vi "LJStreamUD.vi"() -> ()   [LabVIEW 2021]
uses:
  sub/LJstreamUD globals.vi
panel:
  in  "Change Working Directory":bool
  in  "SettlingFactor":i32
  in  "Resolution":i32=1
  in  "Max File Size (Bytes)":i32=1048576 min=1 max=2000000000
  in  "Graph?":bool[](array[boolean])
  out "Address":string
  in  "Disable Scaling":bool
  out "Device Type":string
  in  "stop stream":bool
  in  "exit":bool
  in  "Graph History":i32=1000 min=0
  out "Channel Config":T1={"# Channels"=4, "+Ch"=["0", "1", "2", "3", "4", "5", "6", "7"], "-Ch (U3)"=["31", "31", "31", "31", "31", "31", "31", "31"], "Ranges (UE9)"=[0, 0, 0, 0, 0, 0, 0, 0], "Scaling Equation"=["y=v0", "y=v1", "y=v2", "y=v3", "y=v4", "y=v5", "y=v6", "y=v7"]} {"Ranges (UE9)" items=["LJ_rgBIP5V", "LJ_rgUNI5V", "LJ_rgUNI2P5V", "LJ_rgUNI1P25V", "LJ_rgUNIP625V"]}
  out "Scaled":dbl[](array[numeric]) format="%.6f"
  in  "Scaling Equation":string[](array[string])=["y=v0", "y=v1", "y=v2", "y=v3", "y=v4", "y=v5", "y=v6", "y=v7"]
  in  "# Channels":i32=4 min=1
  in  "-Ch":string[](array[string])=["199", "199", "199", "199", "199", "199", "199", "199"]
  out "Voltage":dbl[](array[numeric]) format="%.6f"
  in  "Ranges":u16[](array[ring])=[0, 0, 0, 0, 0, 0, 0, 0] items=["LJ_rgBIP10V", "LJ_rgBIP5V", "LJ_rgUNI5V", "LJ_rgUNI2P5V", "LJ_rgUNI1P25V", "LJ_rgBIP1V", "LJ_rgUNIP625V", "LJ_rgBIPP1V", "LJ_rgBIPP01V"]
  out "Waveform Graph":cluster{dbl, dbl, dbl[][]}(graph)
  out "UD Backlog [%]":dbl format="%.2f"
  in  "+Ch":string[](array[string])=["0", "1", "2", "3", "4", "5", "6", "7"]
  out "ms Per Loop":u32
  out "Device Backlog [%]":dbl format="%.2f"
  out "# Scans Read":i32
  out "# of iterations":i32
  in  "Scan Rate (Hz)":dbl=500.0 format="%.3f"
  out "Current Data File":path
  in  "Data File Prefix":string="data"
  in  "Write To File":bool
  in  "start stream":bool caption="Start Stream"
  out "Last Stream Error Message":string
  # "0"
  # "1"
  # "2"
  # "3"
  # "4"
  # "5"
  # "6"
  # "7"
  # "8"
  # "9"
  # "10"
  # "11"
  # "12"
  # "13"
  # "14"
  # "15"
  # "Scaling is computing intensive.  If UD Backlog\n  is growing, disable scaling."
  # "# scans"
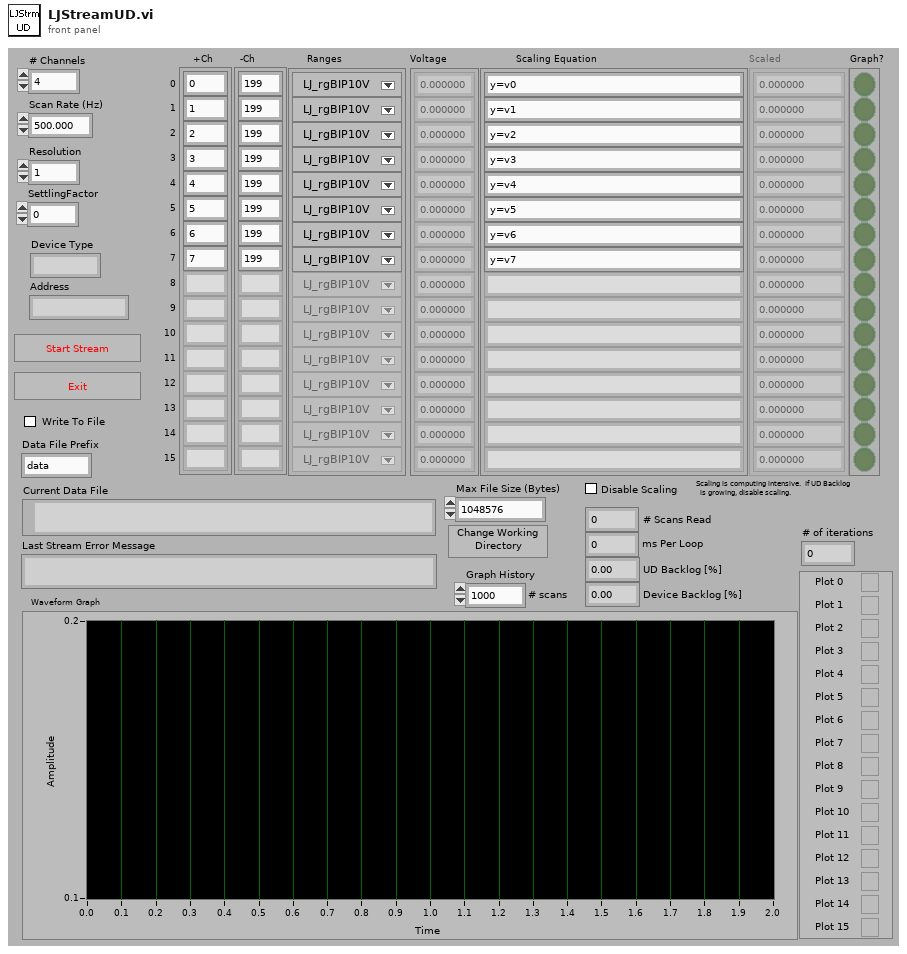
[diagram p1: front panel]
types:
  T1 = cluster{"# Channels":i32, "+Ch":string[], "-Ch (U3)":string[], "Ranges (UE9)":u16[], "Scaling Equation":string[]}
  T2 = cluster{"+Ch":string[], "-Ch":string[], "Ranges":u16[], "Scaling Equation":string[], "Graph?":bool[]}
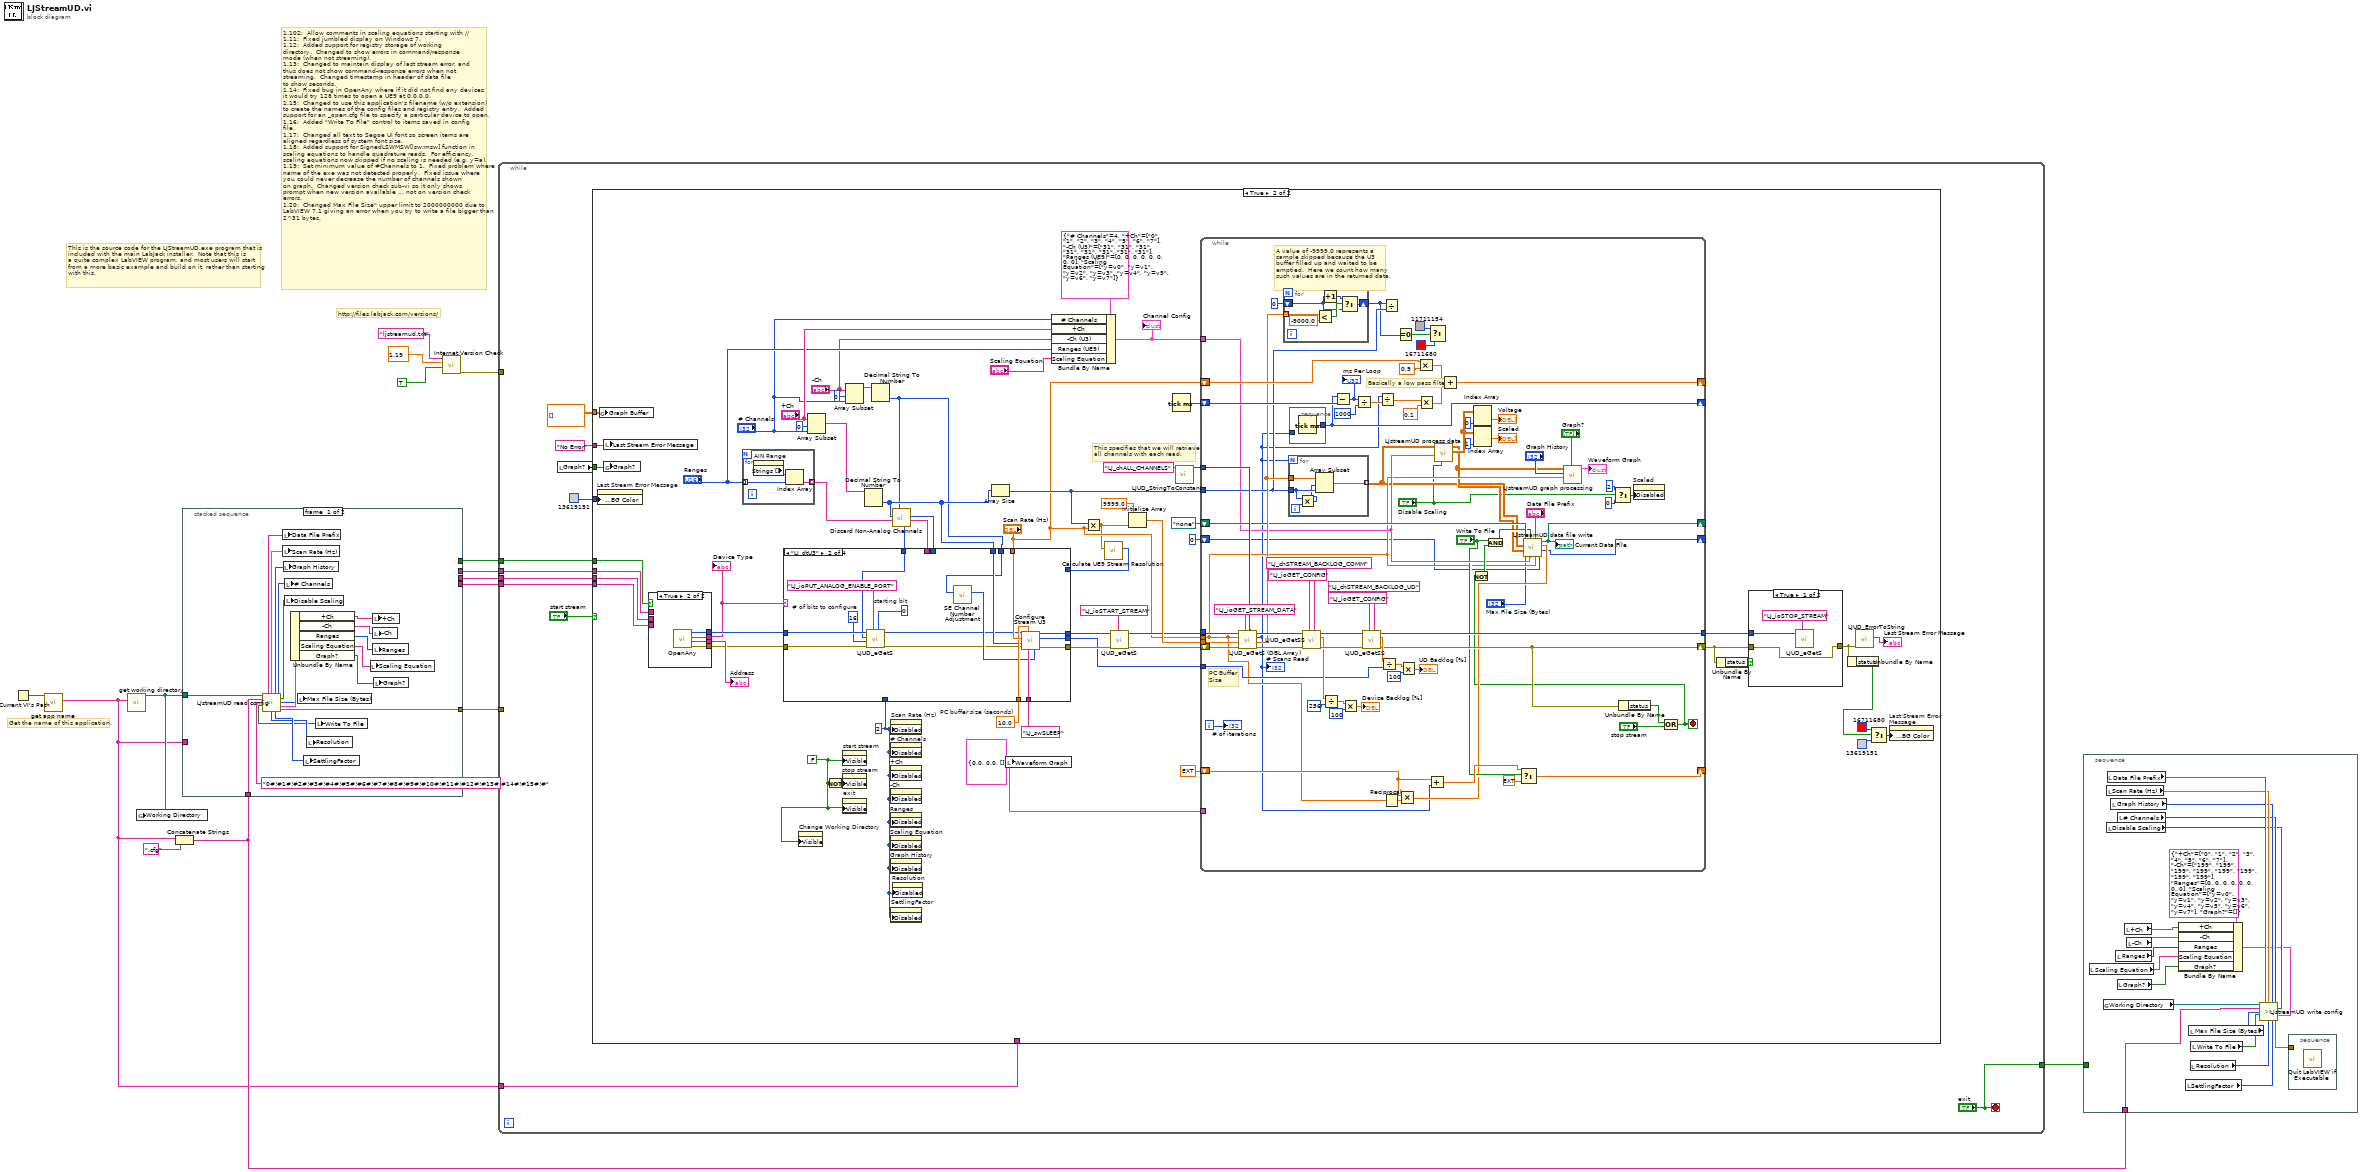
[diagram p0: block diagram]
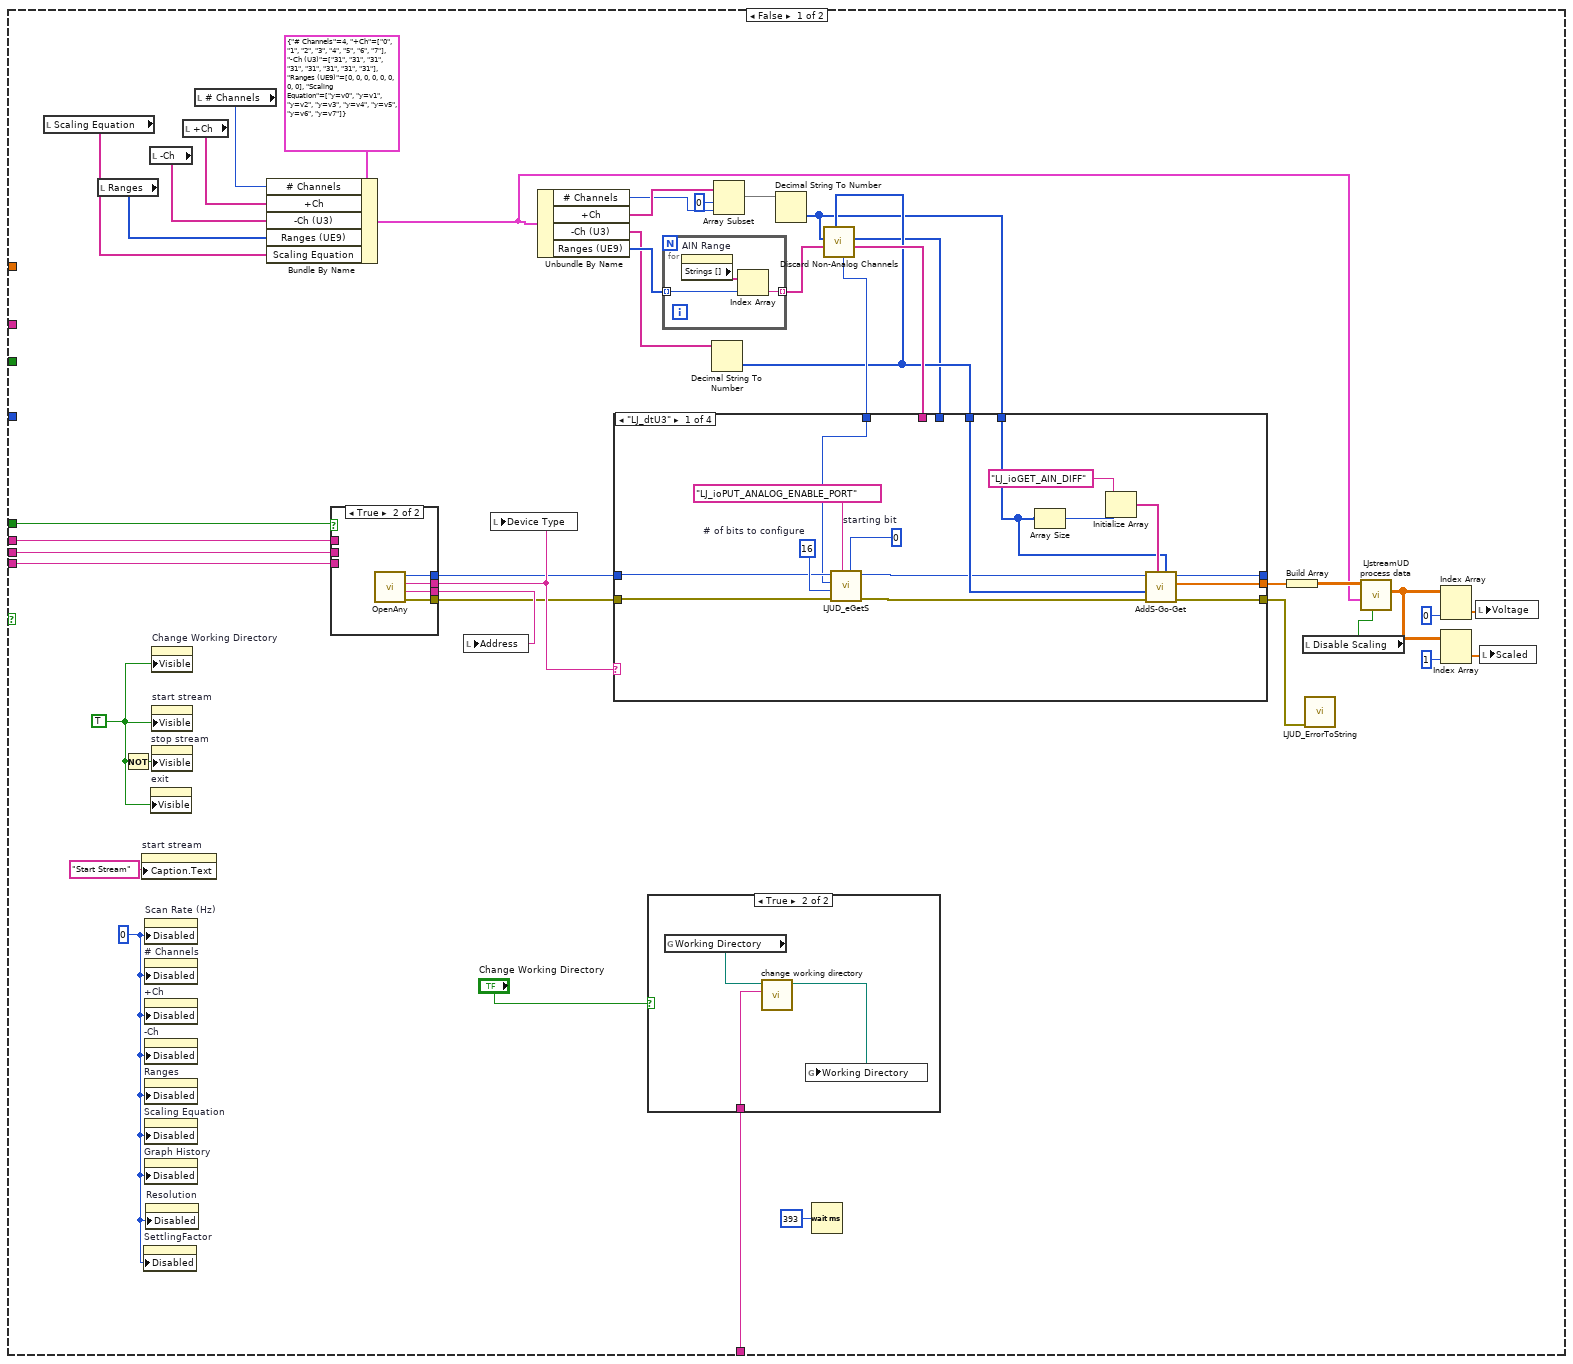
[diagram p2: hidden frame]
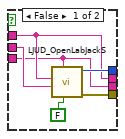
[diagram p3: hidden frame]
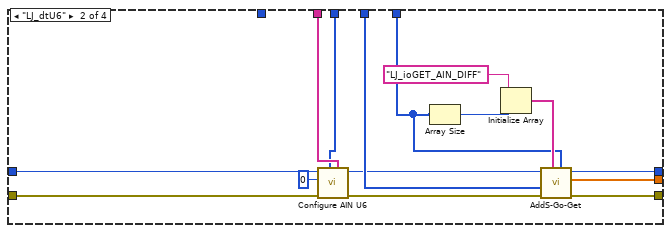
[diagram p5: hidden frame]
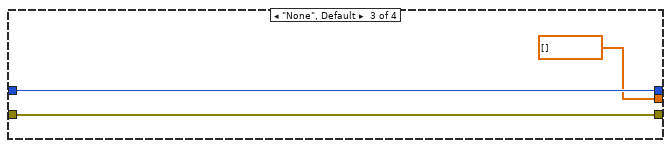
[diagram p6: hidden frame]
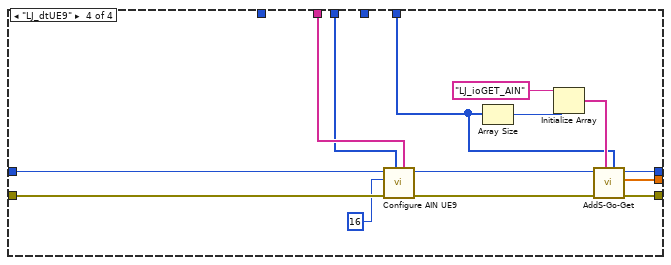
[diagram p7: hidden frame]
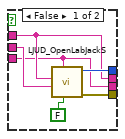
[diagram p8: hidden frame]
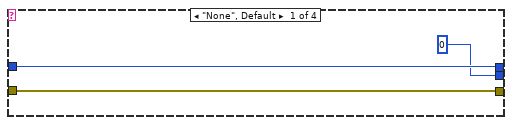
[diagram p9: hidden frame]
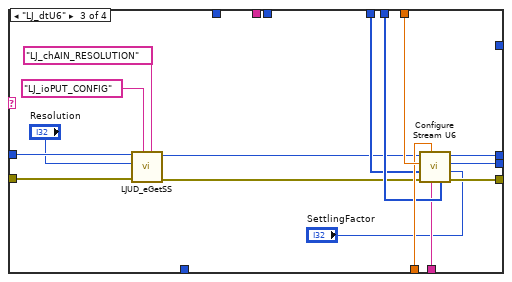
[diagram p10: hidden frame]
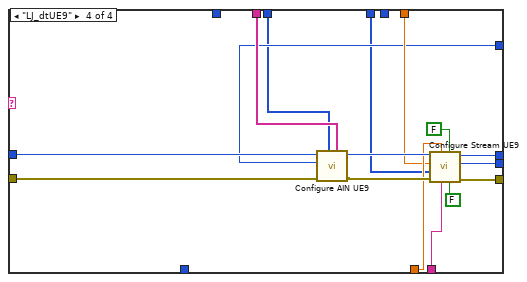
[diagram p11: hidden frame]
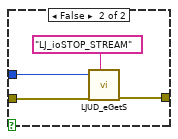
[diagram p12: hidden frame]
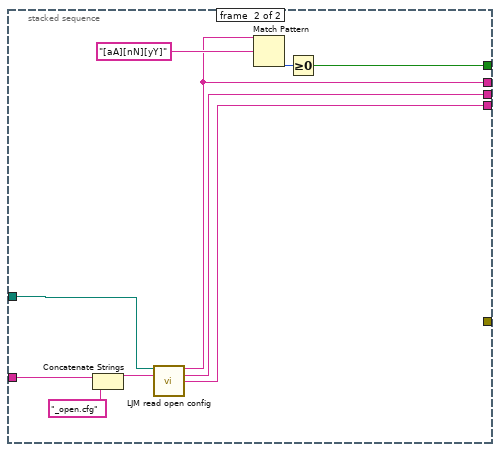
[diagram p13: hidden frame]
diagram:
  # "This is the source code for the LJStreamUD.exe program that is\nincluded with the main LabJack installer.  Note that this is \na quite complex LabVIEW program, and most users will start\nfrom a more basic example and build on it, rather than starting\nwith this."
  # "Get the name of this application."
  # "1.102:  Allow comments in scaling equations starting with //\n1.11:  Fixed jumbled display on Windows 7.\n1.12:  Added support for registry storage of working\ndirectory.  Changed to show errors in command/response\nmode (when not streaming).\n1.13:  Changed to maintain display of last stream error, and\nthus does not show command-response errors when not\nstreaming.  Changed timestamp in header of data file\nto show seconds.\n1.14:  Fixed bug in OpenAny where if it did not find any devices\nit would try 128 times to open a UE9 at 0.0.0.0.\n1.15:  Changed to use this application's filename (w/o extension)\nto create the names of the config files and registry entry.  Added\nsupport for an _open.cfg file to specify a particular device to open.\n1.16:  Added \"Write To File\" control to items saved in config\nfile.\n1.17:  Changed all text to Segoe UI font so screen items are\naligned regardless of system font size.\n1.18:  Added support for SignedLSWMSW[lsw:msw] function in\nscaling equations to handle quadrature reads.  For efficiency,\nscaling equations now skipped if no scaling is needed (e.g. y=a).\n1.19:  Set minimum value of #Channels to 1.  Fixed problem where\nname of the exe was not detected properly.  Fixed issue where\nyou could never decrease the number of channels shown\non graph.  Changed version check sub-vi so it only shows\nprompt when new version available ... not on version check\nerrors.\n1.20:  Changed Max File Size\" upper limit to 2000000000 due to\nLabVIEW 7.1 giving an error when you try to write a file bigger than\n2^31 bytes."
  # "http://files.labjack.com/versions/"
  n1 = Current VI's Path() -> (path=w1:path)
  n2 = call "get app name.vi"("Current VI's Path"=w1) -> ("App Name Without Extension"=w2:string)  [unwired: 4 in, 2 out]
  n3 = call "get working directory.vi"("Application Name"=w2) -> ("Working Directory"=w9:path)  [unwired: 9 in, 1 out]
  n4 = global write "LJstreamUD globals.vi" "Working Directory"(w9) -> ()
  n5 = Concatenate Strings(w2, ".cfg" ("filename")) -> (w7:string)
  n6 = stacked-sequence {
    tunnel: [w34 _] -> w11
    tunnel: w9 -> [w19 w40]
    tunnel: w7 -> [w18 _]
    tunnel: w2 -> [_ w35]
    tunnel: [_ w39] -> w6
    tunnel: [_ w38] -> w5
    tunnel: [_ w37] -> w4
    tunnel: [_ w36] -> w3
    frame #0 {
      n7 = call "LJstreamUD read config.vi"("Working Directory"=w19, "filename"=w18, "ChP Default"="0#!#1#!#2#!#3#!#4#!#5#!#6#!#7#!#8#!#9#!#10#!#11#!#12#!#13#!#14#!#15#!#") -> ("Data File Prefix"=w27:string, "Scan Rate (Hz)"=w26:dbl, "Graph History"=w25:i32, "# Channels"=w24:i32, "Disable Scaling"=w23:bool, "Max File Size (Bytes)"=w22:i32, "Write To File"=w16:bool, "Channel Setup"=w33:T2, "Resolution"=w20:u8, "SettlingFactor"=w21:u8, "error out"=w34:errorcluster)  [unwired: 1 in, 1 out]
      n8 = local write "Data File Prefix"(w27) -> ()
      n9 = local write "Scan Rate (Hz)"(w26) -> ()
      n10 = local write "Graph History"(w25) -> ()
      n11 = local write "# Channels"(w24) -> ()
      n12 = local write "Disable Scaling"(w23) -> ()
      n13 = Unbundle By Name(w33) -> ("+Ch"=w32:string[], "-Ch"=w31:string[], "Ranges"=w30:u16[], "Scaling Equation"=w29:string[], "Graph?"=w28:bool[])
      n14 = local write "Max File Size (Bytes)"(w22) -> ()
      n15 = local write "SettlingFactor"(w21) -> ()
      n16 = local write "Resolution"(w20) -> ()
      n17 = local write "Write To File"(w16) -> ()
      n18 = local write "Scaling Equation"(w29) -> ()
      n19 = local write "+Ch"(w32) -> ()
      n20 = local write "-Ch"(w31) -> ()
      n21 = local write "Ranges"(w30) -> ()
      n22 = local write "Graph?"(w28) -> ()
    }
    frame #1 {
      n23 = Concatenate Strings(w35, "_open.cfg" ("filename")) -> (w42:string)
      n24 = call "LJM read open config.vi"("Working Directory"=w40, "filename"=w42) -> ("DeviceType"=w38:string, "ConnectionType"=w37:string, "Identifier"=w36:string)  [unwired: 10 in, 1 out]
      n25 = Match Pattern(string=w38, regular expression="[aA][nN][yY]") -> (offset past match=w43:i32)  [unwired: 1 in, 3 out]
      n26 = Greater Or Equal To 0?(x=w43) -> (x >= 0?=w39:bool)
    }
  }
  n27 = call "Internet Version Check.vi"("Prompt If Newer Version Available"=TRUE, "Version In"=1.19, "Version File Name"="ljstreamud.txt") -> ("error out"=w12:errorcluster)  [unwired: 6 in, 2 out]
  n28 = while {
    tunnel: w2 -> [w49]
    tunnel: w12 -> [_]
    tunnel: w11 -> [_]
    tunnel: ["exit"] -> w10
    tunnel: w6 -> [w48]
    tunnel: w5 -> [w47]
    tunnel: w4 -> [w46]
    tunnel: w3 -> [w45]
    stop <- "exit" stop-if-true
    n29 = local read "Graph?"() -> (w51:bool[])
    n30 = case shown="True" "start stream" {
      tunnel: "No Error" ("Error Message") -> [_ w190]
      tunnel: dbl[][] [] ("Graph Buffer") -> [_ w182]
      tunnel: w51 -> [_ w181]
      tunnel: u32 13619151 -> [_ w173]
      tunnel: w49 -> [w61 _]
      tunnel: w48 -> [w59 w167]
      tunnel: w47 -> [w58 w166]
      tunnel: w46 -> [w57 w165]
      tunnel: w45 -> [w56 w164]
      frame False {
        w63 = TRUE ("Visible")
        w64 = u8 0 ("Disabled")
        n31 = local read "Scaling Equation"() -> (w70:string[])
        n32 = local read "Ranges"() -> (w71:u16[])
        n33 = Not(x=w63) -> (.not. x?=w97:bool)
        n34 = property on="start stream" class="Bool"("Caption.Text"="Start Stream") -> ()  [unwired: 2 in, 2 out]
        n35 = property on="SettlingFactor" class="DigNum (strict)"("Disabled"=w64) -> ()  [unwired: 2 in, 2 out]
        n36 = property on="Scan Rate (Hz)" class="DigNum (strict)"("Disabled"=w64) -> ()  [unwired: 2 in, 2 out]
        n37 = property on="# Channels" class="DigNum (strict)"("Disabled"=w64) -> ()  [unwired: 2 in, 2 out]
        n38 = property on="+Ch" class="Arr (strict)"("Disabled"=w64) -> ()  [unwired: 2 in, 2 out]
        n39 = property on="-Ch" class="Arr (strict)"("Disabled"=w64) -> ()  [unwired: 2 in, 2 out]
        n40 = property on="Ranges" class="Arr (strict)"("Disabled"=w64) -> ()  [unwired: 2 in, 2 out]
        n41 = property on="Scaling Equation" class="Arr (strict)"("Disabled"=w64) -> ()  [unwired: 2 in, 2 out]
        n42 = property on="Graph History" class="DigNum (strict)"("Disabled"=w64) -> ()  [unwired: 2 in, 2 out]
        n43 = property on="Resolution" class="DigNum (strict)"("Disabled"=w64) -> ()  [unwired: 2 in, 2 out]
        n44 = local read "-Ch"() -> (w72:string[])
        n45 = property on="exit" class="Bool"("Visible"=w63) -> ()  [unwired: 2 in, 2 out]
        n46 = property on="Change Working Directory" class="Bool"("Visible"=w63) -> ()  [unwired: 2 in, 2 out]
        n47 = property on="start stream" class="Bool"("Visible"=w63) -> ()  [unwired: 2 in, 2 out]
        n48 = property on="stop stream" class="Bool"("Visible"=w97) -> ()  [unwired: 2 in, 2 out]
        n49 = local read "+Ch"() -> (w73:string[])
        n50 = local read "# Channels"() -> (w74:i32)
        n51 = Bundle By Name(cluster=T1 {"# Channels"=4, "+Ch"=["0", "1", "2", "3", "4", "5", "6", "7"], "-Ch (U3)"=["31", "31", "31", "31", "31", "31", "31", "31"], "Ranges (UE9)"=[0, 0, 0, 0, 0, 0, 0, 0], "Scaling Equation"=["y=v0", "y=v1", "y=v2", "y=v3", "y=v4", "y=v5", "y=v6", "y=v7"]} ("Channel Config"), "# Channels"=w74, "+Ch"=w73, "-Ch (U3)"=w72, "Ranges (UE9)"=w71, "Scaling Equation"=w70) -> (w75:T1)
        n52 = case shown="True" w59 {
          tunnel: [w101 w108] -> w78
          tunnel: [w99 w107] -> w77
          tunnel: [w104 w106] -> w68
          tunnel: [w103 w105] -> w67
          tunnel: w58 -> [w101 _]
          tunnel: w57 -> [w100 _]
          tunnel: w56 -> [w99 _]
          frame False {
            n53 = call "LJUD_OpenLabJackS.vi"("FirstFound"=FALSE, "Address"=w99, "ConnectionType"=w100, "DeviceType"=w101) -> ("error out"=w103:errorcluster, "Handle"=w104:i32)  [unwired: 5 in, 1 out]
          }
          frame True {
            n54 = call "OpenAny.vi"() -> ("error out"=w105:errorcluster, "Address Found"=w107:string, "Device Type Found"=w108:string, "Handle"=w106:i32)  [unwired: 8 in]
          }
        }
        n55 = local write "Address"(w77) -> ()
        n56 = local write "Device Type"(w78) -> ()
        n57 = Unbundle By Name(w75) -> ("# Channels"=w93:i32, "+Ch"=w94:string[], "-Ch (U3)"=w80:string[], "Ranges (UE9)"=w91:u16[])
        n58 = case shown="True" "Change Working Directory" {
          tunnel: w61 -> [_ w109]
          frame False {
          }
          frame True {
            n59 = global read "LJstreamUD globals.vi" "Working Directory"() -> (w111:path)
            n60 = call "change working directory.vi"("Application Name"=w109, "Working Directory In"=w111) -> ("Working Directory Out"=w110:path)  [unwired: 9 in]
            n61 = global write "LJstreamUD globals.vi" "Working Directory"(w110) -> ()
          }
        }
        n62 = for {
          tunnel: w91 -> [w113] mode=indexing
          tunnel: [w112] -> w90 mode=indexing
          n63 = property on="AIN Range" class="Ring (strict)"() -> ("Strings []"=w114:string[])  [unwired: 2 in, 2 out]
          n64 = Index Array(array=w114, index=w113) -> (element=w112:string)
        }
        n65 = Decimal String To Number(string=w80) -> (number=w79:i32[])  [unwired: 2 in, 1 out]
        n66 = Array Subset(array=w94, index=0 ("Array Index"), length=w93) -> (w92:string[])
        n67 = Decimal String To Number(string=w92) -> (number=w65:i32[])  [unwired: 2 in, 1 out]
        n68 = Wait (ms)(milliseconds to wait=u32 393) -> ()  [unwired: 1 out]
        n69 = call "Discard Non-Analog Channels.vi"("Channels In (-)"=w79, "Ranges In"=w90, "Channels In"=w65) -> ("Ranges Out"=w89:string[], "Channels Out"=w66:i32[], "FIO/EIO Analog Enable"=w88:i32)  [unwired: 5 in, 1 out]
        n70 = case shown="\"LJ_dtU3\"" w78 {
          tunnel: w88 -> [w116 _ _ _]
          tunnel: w67 -> [w120 w133 w147 w161]
          tunnel: w68 -> [w119 w134 w148 w162]
          tunnel: w89 -> [_ w135 _ w160]
          tunnel: w66 -> [_ w132 _ w150]
          tunnel: [w126 w141 w148 w153] -> _
          tunnel: [w127 w142 w147 w152] -> w60
          tunnel: [w125 w140 dbl[] [] ("Values Read") w151] -> w87
          tunnel: w79 -> [w124 w139 _ _]
          tunnel: w65 -> [w115 w131 _ w149]
          frame "LJ_dtU3" {
            w123 = 0  # starting bit
            w121 = 16  # # of bits to configure
            n71 = call "LJUD_eGetS.vi"("Channel"=w123, "IOType"="LJ_ioPUT_ANALOG_ENABLE_PORT" ("Channel"), "error in"=w120, "x1"=w121, "Value Write"=w116, "Handle In"=w119) -> ("error out"=w118:errorcluster, "Handle Out"=w117:i32)  [unwired: 3 in, 1 out]
            n72 = Array Size(array=w115) -> (size(s)=w129:i32)
            n73 = Initialize Array("LJ_ioGET_AIN_DIFF" ("IOType"), w129) -> (w130:string[])
            n74 = call "AddS-Go-Get.vi"("Channels"=w115, "IOTypes"=w130, "error in"=w118, "x1"=w124, "Handle In"=w117) -> ("error out"=w127:errorcluster, "Values Read"=w125:dbl[], "Handle Out"=w126:i32)  [unwired: 4 in]
          }
          frame "LJ_dtU6" {
            n75 = call "Configure AIN U6.vi"("Ranges"=w135, "Positive Channels"=w132, "error in"=w133, "Resolution"=0, "Handle In"=w134) -> ("error out"=w138:errorcluster, "Handle Out"=w137:i32)  [unwired: 5 in]
            n76 = Array Size(array=w131) -> (size(s)=w144:i32)
            n77 = Initialize Array("LJ_ioGET_AIN_DIFF" ("IOType"), w144) -> (w145:string[])
            n78 = call "AddS-Go-Get.vi"("Channels"=w131, "IOTypes"=w145, "error in"=w138, "x1"=w139, "Handle In"=w137) -> ("error out"=w142:errorcluster, "Values Read"=w140:dbl[], "Handle Out"=w141:i32)  [unwired: 4 in]
          }
          frame "None", Default {
          }
          frame "LJ_dtUE9" {
            n79 = call "Configure AIN UE9.vi"("Ranges"=w160, "Channels"=w150, "error in"=w161, "Resolution"=16, "Handle In"=w162) -> ("error out"=w154:errorcluster, "Handle Out"=w155:i32)  [unwired: 5 in]
            n80 = Array Size(array=w149) -> (size(s)=w157:i32)
            n81 = Initialize Array("LJ_ioGET_AIN" ("IOType"), w157) -> (w158:string[])
            n82 = call "AddS-Go-Get.vi"("Channels"=w149, "IOTypes"=w158, "error in"=w154, "Handle In"=w155) -> ("error out"=w152:errorcluster, "Values Read"=w151:dbl[], "Handle Out"=w153:i32)  [unwired: 5 in]
          }
        }
        n83 = Build Array(w87) -> (w86:dbl[][])
        n84 = local read "Disable Scaling"() -> (w69:bool)
        n85 = call "LJUD_ErrorToString.vi"("error in"=w60) -> ()  [unwired: 10 in, 1 out]
        n86 = call "LJstreamUD process data.vi"("Disable Scaling"=w69, "Channel Config"=w75, "Voltages"=w86) -> ("Volts,Scaled Averages"=w83:dbl[][])  [unwired: 7 in, 1 out]
        n87 = Index Array(array=w83, index (col)=0 ("Disabled Index (col)")) -> (element=w82:dbl[])  [unwired: 1 in]
        n88 = Index Array(array=w83, index (col)=1 ("Disabled Index (col)")) -> (element=w81:dbl[])  [unwired: 1 in]
        n89 = local write "Voltage"(w82) -> ()
        n90 = local write "Scaled"(w81) -> ()
      }
      frame True {
        w172 = FALSE ("Visible")
        w179 = u8 2 ("Disabled")
        w192 = cluster{dbl, dbl, dbl[][]} {0.0, 0.0, []} ("Waveform Graph")
        w209 = 10.0  # PC buffer size (seconds)
        # "This specifies that we will retrieve\nall channels with each read."
        n91 = property on="Last Stream Error Message" class="Str"("Text.Text Colors:BG Color"=w173) -> ()  [unwired: 2 in, 2 out]
        n92 = global write "LJstreamUD globals.vi" "Graph Buffer"(w182) -> ()
        n93 = local write "Last Stream Error Message"(w190) -> ()
        n94 = global write "LJstreamUD globals.vi" "Graph?"(w181) -> ()
        n95 = case shown="True" w167 {
          tunnel: [w227 w234] -> w170
          tunnel: [w225 w233] -> w169
          tunnel: [w230 w232] -> w171
          tunnel: [w229 w231] -> w168
          tunnel: w166 -> [w227 _]
          tunnel: w165 -> [w226 _]
          tunnel: w164 -> [w225 _]
          frame False {
            n96 = call "LJUD_OpenLabJackS.vi"("FirstFound"=FALSE, "Address"=w225, "ConnectionType"=w226, "DeviceType"=w227) -> ("error out"=w229:errorcluster, "Handle"=w230:i32)  [unwired: 5 in, 1 out]
          }
          frame True {
            n97 = call "OpenAny.vi"() -> ("error out"=w231:errorcluster, "Address Found"=w233:string, "Device Type Found"=w234:string, "Handle"=w232:i32)  [unwired: 8 in]
          }
        }
        "Device Type" <- w170
        "Address" <- w169
        n98 = for {
          tunnel: "Ranges" -> [w328] mode=indexing
          tunnel: [w327] -> w204 mode=indexing
          n99 = property on="AIN Range" class="Ring (strict)"() -> ("Strings []"=w329:string[])  [unwired: 2 in, 2 out]
          n100 = Index Array(array=w329, index=w328) -> (element=w327:string)
        }
        n101 = property on="Change Working Directory" class="Bool"("Visible"=w172) -> ()  [unwired: 2 in, 2 out]
        n102 = Array Subset(array="+Ch", index=0 ("Array Index"), length="# Channels") -> (w201:string[])
        n103 = Not(x=w172) -> (.not. x?=w191:bool)
        n104 = property on="start stream" class="Bool"("Visible"=w172) -> ()  [unwired: 2 in, 2 out]
        n105 = property on="stop stream" class="Bool"("Visible"=w191) -> ()  [unwired: 2 in, 2 out]
        n106 = property on="exit" class="Bool"("Visible"=w172) -> ()  [unwired: 2 in, 2 out]
        n107 = Array Subset(array="-Ch", index=0 ("Array Index"), length="# Channels") -> (w185:string[])
        n108 = Decimal String To Number(string=w201) -> (number=w189:i32[])  [unwired: 2 in, 1 out]
        n109 = Decimal String To Number(string=w185) -> (number=w187:i32[])  [unwired: 2 in, 1 out]
        n110 = property on="Scan Rate (Hz)" class="DigNum (strict)"("Disabled"=w179) -> ()  [unwired: 2 in, 2 out]
        n111 = property on="# Channels" class="DigNum (strict)"("Disabled"=w179) -> ()  [unwired: 2 in, 2 out]
        n112 = property on="+Ch" class="Arr (strict)"("Disabled"=w179) -> ()  [unwired: 2 in, 2 out]
        n113 = property on="-Ch" class="Arr (strict)"("Disabled"=w179) -> ()  [unwired: 2 in, 2 out]
        n114 = property on="Ranges" class="Arr (strict)"("Disabled"=w179) -> ()  [unwired: 2 in, 2 out]
        n115 = property on="Scaling Equation" class="Arr (strict)"("Disabled"=w179) -> ()  [unwired: 2 in, 2 out]
        n116 = property on="Graph History" class="DigNum (strict)"("Disabled"=w179) -> ()  [unwired: 2 in, 2 out]
        n117 = property on="SettlingFactor" class="DigNum (strict)"("Disabled"=w179) -> ()  [unwired: 2 in, 2 out]
        n118 = call "Discard Non-Analog Channels.vi"("Channels In (-)"=w187, "Ranges In"=w204, "Channels In"=w189) -> ("Ranges Out"=w203:string[], "Channels Out"=w188:i32[], "FIO/EIO Analog Enable"=w210:i32)  [unwired: 5 in, 1 out]
        n119 = property on="Resolution" class="DigNum (strict)"("Disabled"=w179) -> ()  [unwired: 2 in, 2 out]
        n120 = Array Size(array=w189) -> (size(s)=w221:i32)
        n121 = local write "Waveform Graph"(w192) -> ()
        n122 = Bundle By Name(cluster=T1 {"# Channels"=4, "+Ch"=["0", "1", "2", "3", "4", "5", "6", "7"], "-Ch (U3)"=["31", "31", "31", "31", "31", "31", "31", "31"], "Ranges (UE9)"=[0, 0, 0, 0, 0, 0, 0, 0], "Scaling Equation"=["y=v0", "y=v1", "y=v2", "y=v3", "y=v4", "y=v5", "y=v6", "y=v7"]} ("Channel Config"), "# Channels"="# Channels", "+Ch"="+Ch", "-Ch (U3)"="-Ch", "Ranges (UE9)"="Ranges", "Scaling Equation"="Scaling Equation") -> (w197:T1)
        "Channel Config" <- w197
        n123 = Multiply(x=w221, y="Scan Rate (Hz)") -> (x*y=w200:dbl)
        n124 = call "Calculate UE9 Stream Resolution.vi"("Sample Rate"=w200) -> ("Resolution"=w199:i32)  [unwired: 10 in]
        n125 = case shown="\"LJ_dtU3\"" w170 {
          tunnel: "Scan Rate (Hz)" -> [_ w349 w365 w370]
          tunnel: w210 -> [_ w334 _ _]
          tunnel: w168 -> [w332 w339 w356 w374]
          tunnel: w171 -> [w331 w337 w357 w375]
          tunnel: w209 -> [_ w348 w364 w373]
          tunnel: w187 -> [_ w341 w363 _]
          tunnel: w189 -> [_ w347 w362 w367]
          tunnel: [w332 w346 w361 w376] -> w208
          tunnel: [w331 w345 w360 w377] -> w207
          tunnel: [0 ("PC buffer size (samples)") w344 w359 w371] -> w206
          tunnel: "LJ_swSLEEP" ("Wait Mode (2)") -> [_ w343 w358 w372]
          tunnel: w203 -> [_ _ _ w369]
          tunnel: w199 -> [_ _ _ w368]
          tunnel: w179 -> [_ _ _ _]
          tunnel: w188 -> [_ _ _ w366]
          frame "None", Default {
          }
          frame "LJ_dtU3" {
            w333 = 16  # # of bits to configure
            w335 = 0  # starting bit
            n126 = call "LJUD_eGetS.vi"("Channel"=w335, "IOType"="LJ_ioPUT_ANALOG_ENABLE_PORT" ("Channel"), "error in"=w339, "x1"=w333, "Value Write"=w334, "Handle In"=w337) -> ("error out"=w338:errorcluster, "Handle Out"=w336:i32)  [unwired: 3 in, 1 out]
            n127 = call "SE Channel Number Adjustment.vi"("Channels In"=w341) -> ("Channels Out"=w342:i32[])  [unwired: 10 in]
            n128 = call "Configure Stream U3.vi"("Scan List (-)"=w342, "Wait Mode"=w343, "PC buffer size (seconds)"=w348, "error in"=w338, "Scan List (+)"=w347, "Scan Rate (Hz)"=w349, "Handle In"=w336) -> ("error out"=w346:errorcluster, "PC buffer size (samples)"=w344:i32, "Handle Out"=w345:i32)  [unwired: 2 in]
          }
          frame "LJ_dtU6" {
            n129 = call "LJUD_eGetSS.vi"("Channel"="LJ_chAIN_RESOLUTION" ("IOType"), "IOType"="LJ_ioPUT_CONFIG", "error in"=w356, "Value Write"="Resolution", "Handle In"=w357) -> ("error out"=w354:errorcluster, "Handle Out"=w355:i32)  [unwired: 4 in, 1 out]
            n130 = call "Configure Stream U6.vi"("SettlingFactor"="SettlingFactor", "Scan List (-)"=w363, "Wait Mode"=w358, "PC buffer size (seconds)"=w364, "error in"=w354, "Scan List (+)"=w362, "Scan Rate (Hz)"=w365, "Handle In"=w355) -> ("error out"=w361:errorcluster, "PC buffer size (samples)"=w359:i32, "Handle Out"=w360:i32)  [unwired: 1 in]
          }
          frame "LJ_dtUE9" {
            n131 = call "Configure AIN UE9.vi"("Ranges"=w369, "Channels"=w366, "error in"=w374, "Resolution"=w368, "Handle In"=w375) -> ("error out"=w379:errorcluster, "Handle Out"=w378:i32)  [unwired: 5 in]
            n132 = call "Configure Stream UE9.vi"("External Scan Trigger"=FALSE, "Scan Clock Output"=FALSE, "Wait Mode"=w372, "PC buffer size (seconds)"=w373, "error in"=w379, "Scan List"=w367, "Scan Rate (Hz)"=w370, "Handle In"=w378) -> ("error out"=w376:errorcluster, "PC buffer size (samples)"=w371:i32, "Handle Out"=w377:i32)  [unwired: 1 in]
          }
        }
        n133 = call "LJUD_eGetS.vi"("IOType"="LJ_ioSTART_STREAM", "error in"=w208, "Handle In"=w207) -> ("error out"=w212:errorcluster, "Handle Out"=w217:i32)  [unwired: 6 in, 1 out]
        n134 = Initialize Array(9999.0, w200) -> (w222:dbl[])
        n135 = Tick Count (ms)() -> (millisecond timer value=w218:u32)
        n136 = call "LJUD_StringToConstant.vi"("String"="LJ_chALL_CHANNELS") -> ("Constant Number"=w213:i32)  [unwired: 9 in, 1 out]
        n137 = while {
          shift-left: u32 0 ("Data File #") -> [w235]
          shift-right: [w236] -> _
          tunnel: w192 -> [_]
          shift-left: ext 0.0 -> [w253]
          shift-right: [w254] -> _
          tunnel: w197 -> [w258]
          tunnel: w206 -> [w279]
          shift-left: w212 -> [w287]
          shift-right: [w268] -> w211
          tunnel: w213 -> [w292]
          shift-left: "Scan Rate (Hz)" -> [w300]
          shift-right: [w297] -> _
          shift-left: w218 -> [w308]
          shift-right: [w305] -> _
          tunnel: [w269] -> w219
          tunnel: w221 -> [w274]
          tunnel: w222 -> [w310]
          tunnel: "Scan Rate (Hz)" -> [w251]
          shift-left: path "none" ("Current Data File Out") -> [w266]
          shift-right: [w267] -> _
          tunnel: w217 -> [w312]
          i -> [w309]
          stop <- w246 stop-if-true
          # "PC Buffer\nSize"
          # "A value of -9999.0 represents a\nsample skipped because the U3\nbuffer filled up and waited to be\nemptied.  Here we count how many\nsuch values are in the returned data."
          # "Basically a low pass filter"
          n138 = call "LJUD_eGetS (DBL Array).vi"("Channel"=w292, "IOType"="LJ_ioGET_STREAM_DATA", "error in"=w287, "DBL Array Write"=w310, "Value"=w251, "Handle In"=w312) -> ("error out"=w295:errorcluster, "DBL Array Read"=w276:dbl[], "Value"=w249:i32, "Handle Out"=w296:i32)  [unwired: 2 in]
          "# Scans Read" <- w249
          n139 = for {
            shift-right: [w315] -> w271
            shift-left: 0 -> [w316]
            tunnel: w276 -> [w319] mode=indexing
            n140 = Less?(x=w319, y=-9000.0) -> (x < y?=w317:bool)
            n141 = Increment(x=w316) -> (x+1=w320:i32)
            n142 = Select(t=w320, s=w317, f=w316) -> (s? t:f=w315:i32)
          }
          n143 = for {
            N: w249 -> [_]
            tunnel: w276 -> [w326]
            tunnel: w274 -> [w325]
            tunnel: [w322] -> w243 mode=indexing
            i -> [w324]
            n144 = Multiply(x=w325, y=w324) -> (x*y=w323:i32)
            n145 = Array Subset(array=w326, index=w323, length=w325) -> (w322:dbl[])
          }
          n146 = stacked-sequence {
            tunnel: w249 -> [_]
            tunnel: [w321] -> w305
            frame #0 {
              n147 = Tick Count (ms)() -> (millisecond timer value=w321:u32)
            }
          }
          n148 = call "LJUD_eGetSS.vi"("Channel"="LJ_chSTREAM_BACKLOG_COMM", "IOType"="LJ_ioGET_CONFIG", "error in"=w295, "Handle In"=w296) -> ("error out"=w288:errorcluster, "Value Read"=w283:dbl, "Handle Out"=w289:i32)  [unwired: 5 in]
          n149 = Divide(x=w283, y=256) -> (x/y=w286:dbl)
          n150 = Subtract(x=w305, y=w308) -> (x-y=w307:u32)
          "ms Per Loop" <- w307
          n151 = Multiply(x=w286, y=100) -> (x*y=→"Device Backlog [%]":dbl)
          n152 = Divide(x=w307, y=u32 1000) -> (x/y=w304:dbl)
          n153 = call "LJUD_eGetSS.vi"("Channel"="LJ_chSTREAM_BACKLOG_UD", "IOType"="LJ_ioGET_CONFIG", "error in"=w288, "Handle In"=w289) -> ("error out"=w268:errorcluster, "Value Read"=w278:dbl, "Handle Out"=w269:i32)  [unwired: 5 in]
          n154 = Divide(x=w249, y=w304) -> (x/y=w303:dbl)
          n155 = Divide(x=w278, y=w279) -> (x/y=w280:dbl)
          n156 = Divide(x=w271, y=w274) -> ()  [unwired: 1 out]
          n157 = Reciprocal(x=w251) -> (1/x=w257:dbl)
          n158 = Equal To 0?(x=w271) -> (x = 0?=w270:bool)
          n159 = Multiply(x=w253, y=w257) -> (x*y=w250:ext)
          n160 = Multiply(x=w280, y=100) -> (x*y=→"UD Backlog [%]":dbl)
          n161 = Multiply(x=w300, y=0.9) -> (x*y=w299:dbl)
          n162 = Multiply(x=w303, y=0.1) -> (x*y=w298:dbl)
          n163 = Add(x=w253, y=w249) -> (x+y=w255:ext)
          n164 = Select(t=u32 11711154, s=w270, f=u32 16711680) -> ()  [unwired: 1 out]
          n165 = call "LJstreamUD process data.vi"("Disable Scaling"="Disable Scaling", "Channel Config"=w258, "Voltages"=w243) -> ("Volts,Scaled Averages"=w245:dbl[][], "Scaled Data"=w244:dbl[][])  [unwired: 7 in]
          n166 = Add(x=w299, y=w298) -> (x+y=w297:dbl)
          n167 = Index Array(array=w245, index (col)=0 ("Disabled Index (col)")) -> (element=→"Voltage":dbl[])  [unwired: 1 in]
          n168 = Index Array(array=w245, index (col)=1 ("Disabled Index (col)")) -> (element=→"Scaled":dbl[])  [unwired: 1 in]
          n169 = Select(t=w255, s="Write To File", f=ext 0.0) -> (s? t:f=w254:ext)
          n170 = call "LJstreamUD graph processing.vi"("Graph?"="Graph?", "Scan Rate"=w251, "Graph History (# scans)"="Graph History", "Scaled Data"=w244) -> ("Graph Data"=→"Waveform Graph":cluster{dbl, dbl, dbl[][]})  [unwired: 7 in]
          n171 = Select(t=u8 2, s="Disable Scaling", f=u8 0) -> (s? t:f=w241:u8)
          n172 = Unbundle By Name(w268) -> ("status"=w247:bool)
          n173 = property on="Scaled" class="Arr (strict)"("Disabled"=w241) -> ()  [unwired: 2 in, 2 out]
          n174 = Compound Arithmetic op=OR(w247, "stop stream") -> (w246:bool)
          n175 = Not(x=w246) -> (.not. x?=w313:bool)
          n176 = And(x="Write To File", y=w313) -> (x .and. y?=w265:bool)
          n177 = call "LJstreamUD data file write.vi"("Starting #"=w235, "Time"=w250, "Scan Rate"=w251, "Data File Prefix"="Data File Prefix", "Channel Config"=w258, "Write To File"=w265, "max file size (bytes)"="Max File Size (Bytes)", "Scaled Data"=w244, "Voltages"=w243, "Current Data File In"=w266) -> ("Data File #"=w236:u32, "Current Data File Out"=w267:path)
          "Current Data File" <- w267
          "# of iterations" <- w309
        }
        n178 = Unbundle By Name(w211) -> ("status"=w215:bool)
        n179 = case shown="True" w215 {
          tunnel: w219 -> [w383 w387]
          tunnel: [w382 w386] -> w176
          tunnel: w211 -> [w382 w385]
          frame True {
            n180 = call "LJUD_eGetS.vi"("IOType"="LJ_ioSTOP_STREAM", "Handle In"=w383) -> ()  [unwired: 7 in, 3 out]
          }
          frame False {
            n181 = call "LJUD_eGetS.vi"("IOType"="LJ_ioSTOP_STREAM", "error in"=w385, "Handle In"=w387) -> ("error out"=w386:errorcluster)  [unwired: 6 in, 2 out]
          }
        }
        n182 = Unbundle By Name(w176) -> ("status"=w175:bool)
        n183 = call "LJUD_ErrorToString.vi"("error in"=w176) -> ("String"=→"Last Stream Error Message":string)  [unwired: 10 in]
        n184 = Select(t=u32 16711680, s=w175, f=u32 13619151) -> (s? t:f=w174:u32)
        n185 = property on="Last Stream Error Message" class="Str"("Text.Text Colors:BG Color"=w174) -> ()  [unwired: 2 in, 2 out]
      }
    }
  }
  n186 = stacked-sequence {
    tunnel: w10 -> [_]
    tunnel: w7 -> [w390]
    frame #0 {
      n187 = local read "Scaling Equation"() -> (w397:string[])
      n188 = global read "LJstreamUD globals.vi" "Working Directory"() -> (w391:path)
      n189 = local read "Scan Rate (Hz)"() -> (w405:dbl)
      n190 = local read "Disable Scaling"() -> (w402:bool)
      n191 = local read "Data File Prefix"() -> (w406:string)
      n192 = local read "Graph History"() -> (w404:i32)
      n193 = local read "Ranges"() -> (w398:u16[])
      n194 = local read "Graph?"() -> (w396:bool[])
      n195 = local read "# Channels"() -> (w403:i32)
      n196 = local read "+Ch"() -> (w400:string[])
      n197 = local read "-Ch"() -> (w399:string[])
      n198 = Bundle By Name(cluster=T2 {"+Ch"=["0", "1", "2", "3", "4", "5", "6", "7"], "-Ch"=["199", "199", "199", "199", "199", "199", "199", "199"], "Ranges"=[0, 0, 0, 0, 0, 0, 0, 0], "Scaling Equation"=["y=v0", "y=v1", "y=v2", "y=v3", "y=v4", "y=v5", "y=v6", "y=v7"], "Graph?"=[]} ("Channel Setup"), "+Ch"=w400, "-Ch"=w399, "Ranges"=w398, "Scaling Equation"=w397, "Graph?"=w396) -> (w395:T2)
      n199 = local read "SettlingFactor"() -> (w393:i32)
      n200 = local read "Max File Size (Bytes)"() -> (w394:i32)
      n201 = local read "Resolution"() -> (w392:i32)
      n202 = local read "Write To File"() -> (w389:bool)
      n203 = call "LJstreamUD write config.vi"("Working Directory"=w391, "Data File Prefix"=w406, "Scan Rate (Hz)"=w405, "Graph History"=w404, "# Channels"=w403, "filename"=w390, "Disable Scaling"=w402, "Max File Size (Bytes)"=w394, "Write To File"=w389, "Channel Setup"=w395, "Resolution"=w392, "SettlingFactor"=w393) -> ("error out"=w407:errorcluster)  [unwired: 3 in]
      n204 = stacked-sequence {
        tunnel: w407 -> [_]
        frame #0 {
          n205 = call "Quit LabVIEW if Executable.vi"() -> ()  [unwired: 1 in]
        }
      }
    }
  }
